vi "Generate Tiff Tags.vi"() -> (2 "sorted array":T4(array[cluster]))   [LabVIEW 2020, in "LV Tiff.lvlib"]
uses:
  LV Tiff.lvlib
  Tiff Data Type.ctl
  6ed87f8e-63f0-4476-abca-e6390ef1575e.vi
  <vilib>/Comparison/Less/Less Functor/Less Functor.lvclass
panel:
  out "Map 2":T2(c390)
  in  "Ring":u16(ring) items=["NewSubFileType"=254, "SubFileType"=255, "ImageWidth"=256, "ImageHeight"=257, "BitsPerSample"=258, "Compression"=259, "PhotometricInterpretation"=262, "Thresholding"=263, "CellWidth"=264, "CellLength"=265, "FillOrder"=266, "DocumentName"=269, "ImageDescription"=270, "Make"=271, "Model"=272, "StripOffsets"=273, "Orientation"=274, "SamplesPerPixel"=277, "RowsPerStrip"=278, "StripByteCounts"=279, "MinSampleValue"=280, "MaxSampleValue"=281, "XResolution"=282, "YResolution"=283, "PlanarConfiguration"=284, "PageName"=285, "XPosition"=286, "YPosition"=287, "FreeOffsets"=288, "FreeByteCounts"=289, "GrayResponseUnit"=290, "GrayResponseCurve"=291, "T4Options[2]"=292, "T6Options[3]"=293, "ResolutionUnit"=296, "PageNumber"=297, "ColorResponseUnit"=300, "TransferFunction[4]"=301, "Software"=305, "DateTime"=306, "Artist"=315, "HostComputer"=316, "Predictor"=317, "WhitePoint"=318, "PrimaryChromaticities"=319, "ColorMap"=320, "HalftoneHints"=321, "TileWidth"=322, "TileLength"=323, "TileOffsets"=324, "TileByteCounts"=325, "BadFaxLines"=326, "CleanFaxData"=327, "ConsecutiveBadFaxLines"=328, "InkSet"=332, "InkNames"=333, "NumberOfInks"=334, "DotRange"=336, "TargetPrinter"=337, "ExtraSamples"=338, "SampleFormat"=339, "SMinSampleValue"=340, "SMaxSampleValue"=341, "TransferRange"=342, "JPEGProc"=512, "JPEGInterchangeFormat"=513, "JPEGInterchangeFormatLength"=514, "JPEGRestartInterval"=515, "JPEGLosslessPredictors"=517, "JPEGPointTransforms"=518, "JPEGQTables"=519, "JPEGDCTTables"=520, "JPEGACTTables"=521, "YCbCrCoefficients"=529, "YCbCrSubSampling"=530, "YCbCrPositioning"=531, "ReferenceBlackWhite"=532, "Copyright"=33432]
  out "Map":T3(c390)
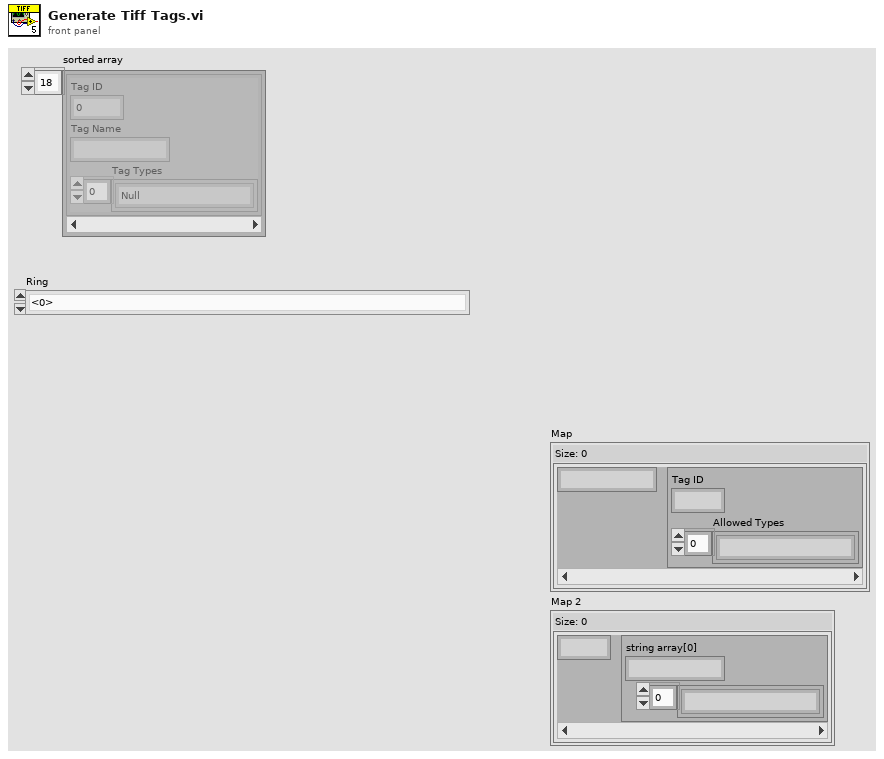
[diagram p1: front panel]
types:
  T1 = typedef "LV Tiff.lvlib/Tiff Data Type.ctl" = enum16{"Null", "BYTE", "ASCII", "SHORT", "LONG", "RATIONAL", "SBYTE", "UNDEFINE", "SSHORT", "SLONG", "SRATIONAL", "FLOAT", "DOUBLE"}
  T2 = map{u16, cluster{"string array[0]":string, T1[]}}
  T3 = map{string, cluster{"Tag ID":u32, "Allowed Types":T1[]}}
  T4 = cluster{"Tag ID":i32, "Tag Name":string, "Tag Types":T1[]}[]
  T5 = cluster{"string array[0]":string, "string array[1]":string, "string array[2]":string}
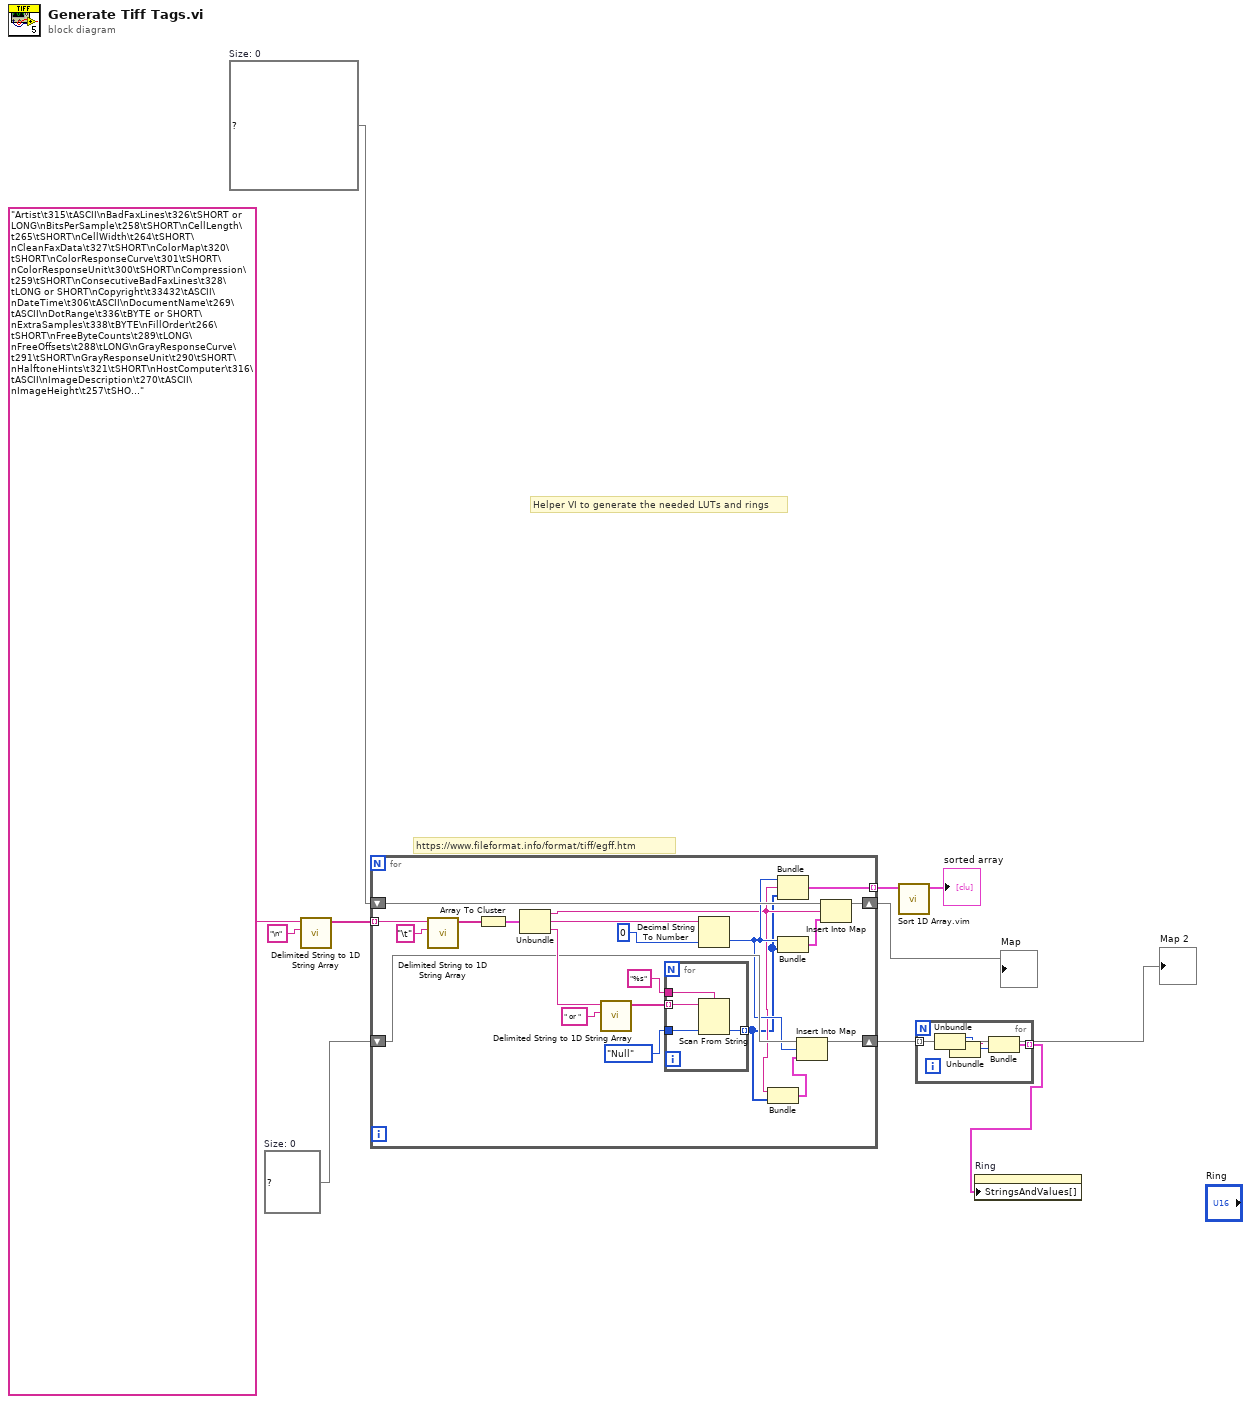
[diagram p0: block diagram]
diagram:
  w3 = T2 {}  # Size: 0
  w5 = T3 {}  # Size: 0
  # "Helper VI to generate the needed LUTs and rings"
  # "https://www.fileformat.info/format/tiff/egff.htm"
  n1 = call <vilib>:"Delimited String to 1D String Array.vi"("delimiter"="\n", "delimited string"="Artist\t315\tASCII\nBadFaxLines\t326\tSHORT or LONG\nBitsPerSample\t258\tSHORT\nCellLength\t265\tSHORT\nCellWidth\t264\tSHORT\nCleanFaxData\t327\tSHORT\nColorMap\t320\tSHORT\nColorResponseCurve\t301\tSHORT\nColorResponseUnit\t300\tSHORT\nCompression\t259\tSHORT\nConsecutiveBadFaxLines\t328\tLONG or SHORT\nCopyright\t33432\tASCII\nDateTime\t306\tASCII\nDocumentName\t269\tASCII\nDotRange\t336\tBYTE or SHORT\nExtraSamples\t338\tBYTE\nFillOrder\t266\tSHORT\nFreeByteCounts\t289\tLONG\nFreeOffsets\t288\tLONG\nGrayResponseCurve\t291\tSHORT\nGrayResponseUnit\t290\tSHORT\nHalftoneHints\t321\tSHORT\nHostComputer\t316\tASCII\nImageDescription\t270\tASCII\nImageHeight\t257\tSHORT or LONG\nImageWidth\t256\tSHORT or LONG\nInkNames\t333\tASCII\nInkSet\t332\tSHORT\nJPEGACTTables\t521\tLONG\nJPEGDCTTables\t520\tLONG\nJPEGInterchangeFormat\t513\tLONG\nJPEGInterchangeFormatLength\t514\tLONG\nJPEGLosslessPredictors\t517\tSHORT\nJPEGPointTransforms\t518\tSHORT\nJPEGProc\t512\tSHORT\nJPEGRestartInterval\t515\tSHORT\nJPEGQTables\t519\tLONG\nMake\t271\tASCII\nMaxSampleValue\t281\tSHORT\nMinSampleValue\t280\tSHORT\nModel\t272\tASCII\nNewSubFileType\t254\tLONG\nNumberOfInks\t334\tSHORT\nOrientation\t274\tSHORT\nPageName\t285\tASCII\nPageNumber\t297\tSHORT\nPhotometricInterpretation\t262\tSHORT\nPlanarConfiguration\t284\tSHORT\nPredictor\t317\tSHORT\nPrimaryChromaticities\t319\tRATIONAL\nReferenceBlackWhite\t532\tLONG\nResolutionUnit\t296\tSHORT\nRowsPerStrip\t278\tSHORT or LONG\nSampleFormat\t339\tSHORT\nSamplesPerPixel\t277\tSHORT\nSMaxSampleValue\t341\tAny\nSMinSampleValue\t340\tAny\nSoftware\t305\tASCII\nStripByteCounts\t279\tLONG or SHORT\nStripOffsets\t273\tSHORT or LONG\nSubFileType\t255\tSHORT\nT4Options[2]\t292\tLONG\nT6Options[3]\t293\tLONG\nTargetPrinter\t337\tASCII\nThresholding\t263\tSHORT\nTileByteCounts\t325\tSHORT or LONG\nTileLength\t323\tSHORT or LONG\nTileOffsets\t324\tLONG\nTileWidth\t322\tSHORT or LONG\nTransferFunction[4]\t301\tSHORT\nTransferRange\t342\tSHORT\nXPosition\t286\tRATIONAL\nXResolution\t282\tRATIONAL\nYCbCrCoefficients\t529\tRATIONAL\nYCbCrPositioning\t531\tSHORT\nYCbCrSubSampling\t530\tSHORT\nYPosition\t287\tRATIONAL\nYResolution\t283\tRATIONAL\nWhitePoint\t318\tRATIONAL") -> ("string array"=w8:string[])  [unwired: 9 in]
  n2 = for {
    tunnel: w8 -> [w31] mode=indexing
    tunnel: [w26] -> w7 mode=indexing
    shift-right: [w19] -> w4
    shift-left: w5 -> [w20]
    shift-right: [w15] -> w2
    shift-left: w3 -> [w16]
    n3 = call <vilib>:"Delimited String to 1D String Array.vi"("delimiter"="\t", "delimited string"=w31) -> ("string array"=w29:string[])  [unwired: 9 in]
    n4 = Array To Cluster(array=w29) -> (cluster=w28:T5)
    n5 = Unbundle(w28) -> ("string array[0]"=w13:string, "string array[1]"=w27:string, "string array[2]"=w23:string)
    n6 = call <vilib>:"Delimited String to 1D String Array.vi"("delimiter"=" or ", "delimited string"=w23) -> ("string array"=w21:string[])  [unwired: 9 in]
    n7 = for {
      tunnel: "%s" ("format string") -> [w34]
      tunnel: w21 -> [w32] mode=indexing
      tunnel: Tiff_Data_Type."Null" ("DataType") -> [w35]
      tunnel: [w33] -> w12 mode=indexing
      n8 = Scan From String(format string=w34, input string=w32, default 1=w35) -> (output 1=w33:T1)  [unwired: 2 in, 3 out]
    }
    n9 = Decimal String To Number(string=w27, default (0L)=u16 0) -> (number=w14:u16)  [unwired: 1 in, 1 out]
    n10 = Bundle("string array[0]"=w13, w12) -> (w11:cluster{"string array[0]":string, T1[]})  [unwired: 1 in]
    n11 = Bundle(w14, "string array[0]"=w13, w12) -> (w26:cluster{u16, "string array[0]":string, T1[]})  [unwired: 1 in]
    n12 = Bundle(w14, w12) -> (w18:cluster{u16, T1[]})  [unwired: 1 in]
    n13 = Insert Into Map(map in=w16, key=w14, value=w11) -> (map out=w15:T2)  [unwired: 2 out]
    n14 = Insert Into Map(map in=w20, key=w13, value=w18) -> (map out=w19:T3)  [unwired: 2 out]
  }
  "Map" <- w4
  "Map 2" <- w2
  n15 = call "Sort 1D Array.vim"("unsorted array"=w7) -> ("sorted array"=→"sorted array":cluster{u16, "string array[0]":string, T1[]}[])  [unwired: 10 in]
  n16 = for {
    tunnel: w2 -> [w40] mode=indexing
    tunnel: [w37] -> w1 mode=indexing
    n17 = Unbundle(w40) -> ("number"=w39:u16, w38:cluster{"string array[0]":string, T1[]})
    n18 = Unbundle(w38) -> ("string array[0]"=w36:string)  [unwired: 1 out]
    n19 = Bundle("string array[0]"=w36, "number"=w39) -> (w37:cluster{"string array[0]":string, "number":u16})  [unwired: 1 in]
  }
  n20 = property on="Ring" class="Ring (strict)"("StringsAndValues[]"=w1) -> ()  [unwired: 2 in, 2 out]
